vi "tripod gait (graph).vi"(0 "data of 5th order formula\nts,tair,a1-a6":dbl[](array[numeric]), 3 "buffer ratio":dbl, 4 "t_shift":dbl=0.000125, 5 "sample time":dbl=0.002, 9 "T_ratio":dbl, 10 "initial":bool) -> (13 "set point":dbl(graph), 14 "now gait info":T1, 23 "Set Point":dbl, 24 "Set Point 2":dbl)   [LabVIEW 2019]
panel:
  in  "Confirm(indicator)":bool
  in  "initial step count":dbl
  out "Confirm":bool
  out "reset cost":bool
  out "start to calculate power":bool
  out "start to calculate the cost":bool
  out "step count NM":dbl
  out "period":dbl
  out "finished":bool
  out "beta":dbl
  out "state":dbl
  out "t2 out":dbl
  out "t1 out":dbl
  # "Nelder Mead"
  # "Input"
  # "Output"
  # "Others"
  # "loop period(ms)"
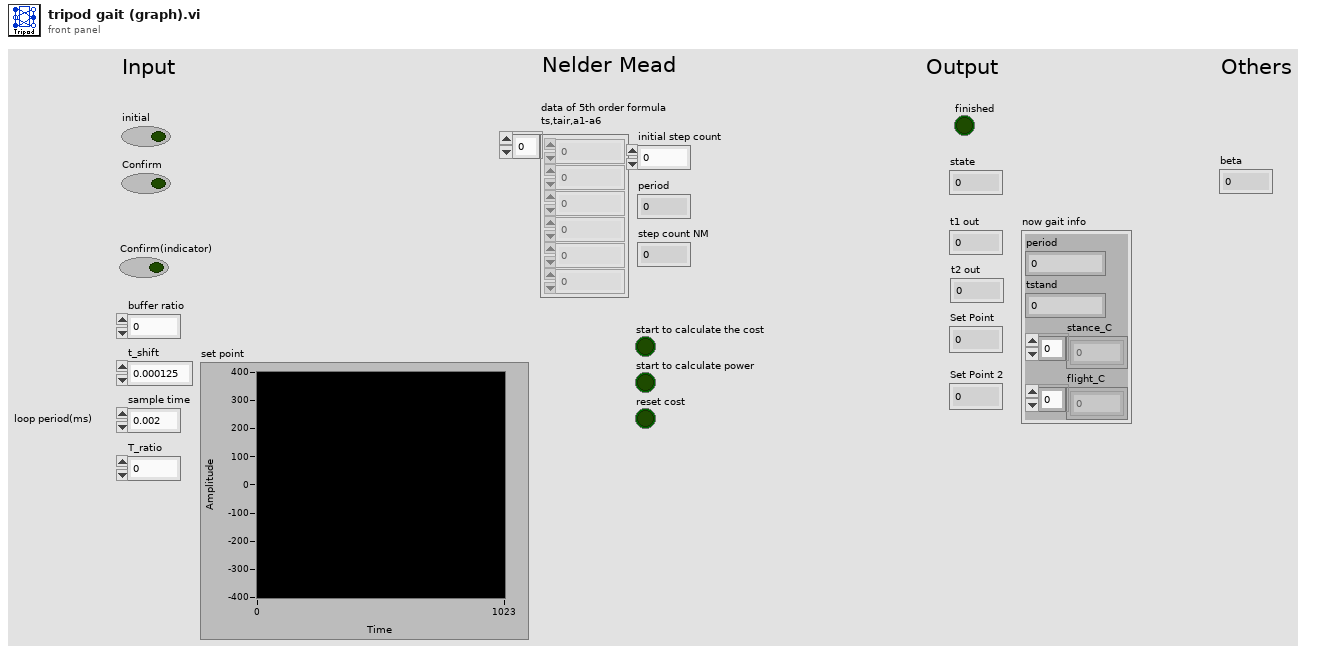
[diagram p1: front panel]
types:
  T1 = cluster{"period":dbl, "tstand":dbl, "stance_C":dbl[], "flight_C":dbl[]}
  T2 = cluster{"output cluster 2":cluster{"period":dbl, "tstand":dbl, "stance_C":dbl[], "flight_C":dbl[]}, "time180":dbl}
  T3 = cluster{"output cluster 2":cluster{"period":dbl, "tstand":dbl, "stance_C":dbl[], "flight_C":dbl[]}, "t2_out":dbl}
  T4 = cluster{"output cluster 2":cluster{"period":dbl, "tstand":dbl, "stance_C":dbl[], "flight_C":dbl[]}, "t1_out":dbl}
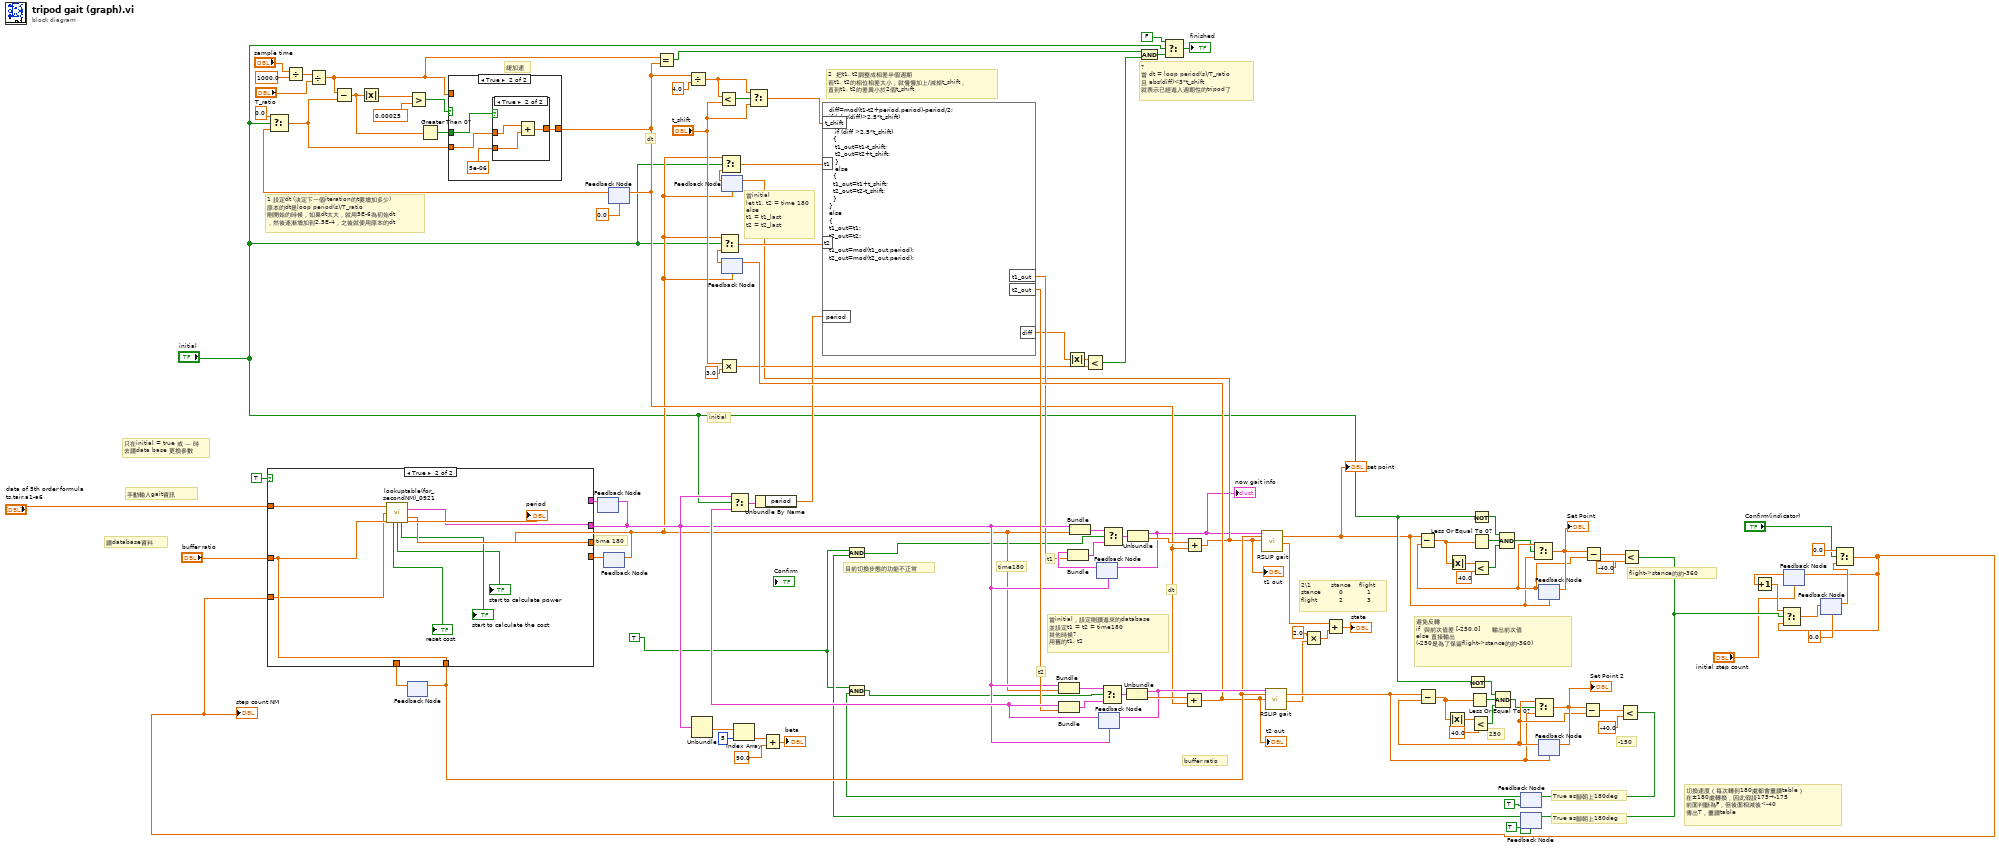
[diagram p0: block diagram]
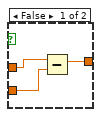
[diagram p3: hidden frame]
diagram:
  w14 = TRUE
  # "目前切換步態的功能不正常"
  # "True as腳朝上180deg"
  # "True as腳朝上180deg"
  # "time180"
  # "t2"
  # "t1"
  # "dt"
  # "當initial，設定剛讀進來的database\n並設定t1 = t2 = time180\n其他時候?\n用舊的t1, t2"
  # "當initial\nlet t1, t2 = time 180\nelse\nt1 = t1_last\nt2 = t2_last"
  # "2  把t1, t2調整成相差半個週期\n若t1, t2的相位相差太小，就慢慢加上/減掉t_shift，\n直到t1, t2的差異小於2個t_shift"
  # "只在initial = true 或 ... 時\n去讀data base 更換參數"
  # "?\n當 dt = loop period(s)/T_ratio\n且 abs(diff)<3*t_shift\n就表示已經進入週期性的tripod了"
  # "1 設定dt (決定下一個iteration的t要增加多少)\n原本的dt是loop period(s)/T_ratio\n剛開始的時候，如果dt太大，就用5E-6為初始dt\n，然後逐漸增加到2.5E-4，之後就使用原本的dt"
  # "dt"
  # "initial"
  # "time 180"
  # "緩加速"
  # "切換速度（每次轉到180處都會重讀table）\n在±180處轉換，因此假設175→-175\n前面判斷為F，但後面相減後<-40\n傳出T，重讀table"
  # "手動輸入gait資訊"
  # "-150"
  # "250"
  # "buffer ratio"
  # "讀database資料"
  # "flight->stance的約-360"
  # "避免反轉\nif  與前次值差 [-250,0]      輸出前次值 \nelse 直接輸出\n(-250是為了保留flight->stance的約-360)"
  # "2\\1          stance    flight\nstance         0            1\nflight           2            3"
  n1 = Divide(x="sample time", y=1000.0) -> (x/y=w49:dbl)
  n2 = Divide(x=w49, y="T_ratio") -> (x/y=w48:dbl)
  n3 = feedback #1() -> (w27:dbl)  [unwired: 1 in]
  n4 = feedback #2() -> (w112:T1)  [unwired: 1 in]
  n5 = feedback #3() -> (w28:dbl)  [unwired: 1 in]
  n6 = feedback #4(0.0 ("sampling time")) -> (w64:dbl)
  n7 = Select(t=0.0, s="initial", f=w64) -> (s? t:f=w63:dbl)
  n8 = Subtract(x=w48, y=w63) -> (x-y=w46:dbl)
  n9 = Absolute Value(x=w46) -> (abs(x)=w68:dbl)
  n10 = Greater?(x=w68, y=0.00025) -> (0:w66:bool)
  n11 = Greater Than 0?(x=w46) -> (x > 0?=w45:bool)
  n12 = case shown="True" w66 {
    tunnel: w48 -> [w114 _]
    tunnel: [w114 w117] -> w54
    tunnel: w63 -> [_ w118]
    tunnel: w45 -> [_ w116]
    frame False {
    }
    frame True {
      n13 = case shown="True" w116 {
        tunnel: w118 -> [w121 w123]
        tunnel: [w120 w124] -> w117
        tunnel: 5e-06 ("x") -> [w119 w122]
        frame False {
          n14 = Subtract(x=w121, y=w119) -> (x-y=w120:dbl)
        }
        frame True {
          n15 = Add(x=w123, y=w122) -> (x+y=w124:dbl)
        }
      }
    }
  }
  n16 = feedback-in #4(w54) -> ()
  n17 = Equal?(x=w48, y=w54) -> (x = y?=w53:bool)
  n18 = Divide(x=w54, y=4.0) -> (x/y=w60:dbl)
  n19 = Less?(x=w60, y="t_shift") -> (x < y?=w61:bool)
  n20 = Multiply(x="t_shift", y=3.0) -> (x*y=w26:dbl)
  n21 = Select(t=w60, s=w61, f="t_shift") -> (s? t:f=w58:dbl)
  n22 = Not(x="initial") -> (.not. x?=w32:bool)
  n23 = Not(x="initial") -> (.not. x?=w36:bool)
  n24 = feedback #5(TRUE) -> (w16:bool)
  n25 = And(x=w14, y=w16) -> (x .and. y?=w20:bool)
  n26 = feedback #6(TRUE) -> (w15:bool)
  n27 = And(x=w14, y=w15) -> (x .and. y?=w19:bool)
  n28 = feedback #7("initial step count") -> (w11:dbl)
  n29 = Increment(x=w11) -> (x+1=w10:dbl)
  n30 = feedback #8(0.0) -> (w12:dbl)
  n31 = Select(t=0.0, s="Confirm(indicator)", f=w12) -> (s? t:f=w2:dbl)
  "step count NM" <- w2
  n32 = case shown="True" TRUE {
    tunnel: "buffer ratio" -> [_ w135]
    tunnel: [w126 w132] -> w25
    tunnel: [w127 w133] -> w71
    tunnel: w112 -> [w127 _]
    tunnel: [w125 w135] -> w75
    tunnel: w28 -> [w126 _]
    tunnel: w27 -> [w125 _]
    tunnel: "data of 5th order formula\nts,tair,a1-a6" -> [_ w136]
    tunnel: w2 -> [_ w128]
    frame False {
    }
    frame True {
      n33 = call "lookuptable(for_secondNM)_0921.vi"("data of 5th order formula\nts,tair,a1-a6 \n(input from the first NM)"=w136, "step count NM"=w128, "buffer ratio"=w135) -> ("output cluster 2"=w133:T1, "time180"=w132:dbl, "reset step(indicator)"=→"reset cost":bool, "start to calculate the power"=→"start to calculate power":bool, "start to calculate the cost"=→"start to calculate the cost":bool, "period"=→"period":dbl)  [unwired: 7 in]
    }
  }
  n34 = feedback-in #1(w75) -> ()
  n35 = feedback-in #2(w71) -> ()
  n36 = feedback-in #3(w25) -> ()
  n37 = Unbundle(w71) -> ("stance_C"=w87:dbl[])  [unwired: 3 out]
  n38 = feedback #9(w25) -> (w39:dbl)
  n39 = Select(t=w25, s="initial", f=w39) -> (s? t:f=w40:dbl)
  n40 = feedback #10(w25) -> (w38:dbl)
  n41 = Select(t=w25, s="initial", f=w38) -> (s? t:f=w37:dbl)
  n42 = Index Array(array=w87, index=5) -> (element=w85:dbl)
  n43 = Add(x=w85, y=90.0) -> (x+y=→"beta":dbl)
  n44 = Bundle("output cluster 2"=w71, "time180"=w25) -> (w98:T2)  [unwired: 1 in]
  n45 = Bundle("output cluster 2"=w71, "time180"=w25) -> (w103:T2)  [unwired: 1 in]
  n46 = feedback #11(w71) -> (w101:T1)
  n47 = feedback #12(w71) -> (w92:T1)
  n48 = Select(t=w71, s="initial", f=w92) -> (s? t:f=w91:T1)
  n49 = Unbundle By Name(w91) -> ("period"=w70:dbl)
  n50 = formula code="diff=mod(t1-t2+period,period)-period/2;\nif (abs(diff)>2.5*t_shift)\n{\n   if (diff >2.5*t_shift)\n  {\n   t1_out=t1-t_shift;\n   t2_out=t2+t_shift;\n   }\n   else \n  {\n  t1_out=t1+t_shift;\n  t2_out=t2-t_shift;\n  }\n}\nelse\n{\nt1_out=t1;\nt2_out=t2;\n}\nt1_out=mod(t1_out,period);\nt2_out=mod(t2_out,period);"("period"=w70, "t1"=w40, "t2"=w37, "t_shift"=w58) -> ("t1_out"=w69:dbl, "t2_out"=w73:dbl, "diff"=w55:dbl)
  n51 = Bundle("output cluster 2"=w92, "t2_out"=w73) -> (w97:T3)  [unwired: 1 in]
  n52 = Absolute Value(x=w55) -> (abs(x)=w56:dbl)
  n53 = Bundle("output cluster 2"=w101, "t1_out"=w69) -> (w100:T4)  [unwired: 1 in]
  n54 = Less?(x=w56, y=w26) -> (x < y?=w52:bool)
  n55 = Select(t=w98, s=w19, f=w97) -> (s? t:f=w99:T3)
  n56 = Select(t=w103, s=w20, f=w100) -> (s? t:f=w102:T4)
  n57 = Unbundle(w99) -> ("output cluster 2"=w78:T1, "t2_out"=w95:dbl)
  n58 = feedback-in #12(w78) -> ()
  n59 = Unbundle(w102) -> ("output cluster 2"=w18:T1, "t1_out"=w96:dbl)
  "now gait info" <- w18
  n60 = feedback-in #11(w18) -> ()
  n61 = And(x=w53, y=w52) -> (x .and. y?=w42:bool)
  n62 = Select(t=FALSE, s="initial", f=w42) -> (s? t:f=→"finished":bool)
  n63 = Add(x=w95, y=w54) -> (x+y=w72:dbl)
  "t2 out" <- w72
  n64 = feedback-in #10(w72) -> ()
  n65 = Add(x=w96, y=w54) -> (x+y=w24:dbl)
  "t1 out" <- w24
  n66 = feedback-in #9(w24) -> ()
  n67 = call "RSLIP gait.vi"("gait Data"=w18, "Buffer Ratio"=w75, "Input Time"=w24) -> ("Set Point"=w1:dbl, "state"=w79:dbl)  [unwired: 13 in, 2 out]
  "set point" <- w1
  n68 = call "RSLIP gait.vi"("gait Data"=w78, "Buffer Ratio"=w75, "Input Time"=w72) -> ("Set Point"=w77:dbl, "state"=w76:dbl)  [unwired: 13 in, 2 out]
  n69 = Multiply(x=2.0, y=w76) -> (x*y=w89:dbl)
  n70 = Add(x=w79, y=w89) -> (x+y=→"state":dbl)
  n71 = feedback #13(w1) -> (w74:dbl)
  n72 = Subtract(x=w1, y=w74) -> (x-y=w109:dbl)
  n73 = Absolute Value(x=w109) -> (abs(x)=w108:dbl)
  n74 = Less Or Equal To 0?(x=w109) -> (x <= 0?=w35:bool)
  n75 = Less?(x=w108, y=40.0) -> (x < y?=w34:bool)
  n76 = Compound Arithmetic op=AND(w36, w35, w34) -> (w33:bool)
  n77 = Select(t=w74, s=w33, f=w1) -> (s? t:f=w93:dbl)
  "Set Point" <- w93
  n78 = feedback-in #13(w93) -> ()
  n79 = feedback #14(w77) -> (w82:dbl)
  n80 = Subtract(x=w77, y=w82) -> (x-y=w107:dbl)
  n81 = Absolute Value(x=w107) -> (abs(x)=w106:dbl)
  n82 = Less Or Equal To 0?(x=w107) -> (x <= 0?=w31:bool)
  n83 = Less?(x=w106, y=40.0) -> (x < y?=w30:bool)
  n84 = Compound Arithmetic op=AND(w32, w31, w30) -> (w29:bool)
  n85 = Select(t=w82, s=w29, f=w77) -> (s? t:f=w94:dbl)
  "Set Point 2" <- w94
  n86 = feedback-in #14(w94) -> ()
  n87 = Subtract(x=w94, y=w82) -> (x-y=w105:dbl)
  n88 = Subtract(x=w93, y=w74) -> (x-y=w111:dbl)
  n89 = Less?(x=w105, y=-40.0) -> (x < y?=w21:bool)
  n90 = feedback-in #6(w21) -> ()
  n91 = Less?(x=w111, y=-40.0) -> (x < y?=w6:bool)
  n92 = feedback-in #5(w6) -> ()
  n93 = Select(t=w10, s=w6, f=w2) -> (s? t:f=w7:dbl)
  n94 = feedback-in #7(w2) -> ()
  n95 = feedback-in #8(w7) -> ()
